vi "AlliGator Compute Phasor Ratio at Mouse Location.vi"(7 "AlliGator Ctrl Refnums":T4, 8 "error in (no error)":errorcluster, 9 "Interactive?":bool, 10 "Mouse Click Event Data":T1, 11 "Data Value Reference in":refnum<data-value>) -> (0 "error out":errorcluster, 1 "Message":string, 3 "Data Value Reference out":refnum<data-value>)   [LabVIEW 2021, in "AlliGator Phasor Ratio.lvlib"]
doc: "Computes phasor ratio and derived quantities at mouse location (interactively or using the last computed phasor) and updates a variety of indicators."
uses:
  AlliGator Phasor Ratio.lvlib
  AlliGator Internal Variables v2.ctl
  <vilib>/vision/Image Controls.llb/IMAQ Image.ctl
  AlliGator Gate Image Set.ctl
  AlliGator FLI Dataset Type.ctl
  AlliGator Data Series Type.ctl
  AlliGator Dataset Channel.ctl
  AlliGator Gate Arithmetic.ctl
  AlliGator Displayed Image.ctl
  Image/Named ROI Description.ctl
  AlliGator Decay Metadata v3.ctl
  AlliGator Decay Background Subtraction Info.ctl
  AlliGator Baseline Subtraction Method.ctl
  Graphs/XY Graph/XY Graph Plot Shift Parameters.ctl
  Graphs/XY Graph/XY Graph Plot Shift Method.ctl
  AlliGator Decay Extrapolation Parameters.ctl
  Phasor/Calibration Phasor (m, phi).ctl
  Phasor/Phasor Reference Series.ctl
  Phasor/Phasor Calibration Map v2.ctl
  Phasor/Phasor (g, s).ctl
  AlliGator Raw Phasor Plot Data v4.ctl
  Phasor/Phasor Standard Deviation Options.ctl
  AlliGator Phasor Multi-Harmonic Data.ctl
  Phasor/Phasor Harmonic Data.ctl
  AlliGator Decay Fit Options & Parameters v2.ctl
  Fits/IRF(X)PSED/Decay Fit Options v2.ctl
  Fits/Decay Convolution/Decay Model.ctl
  Fits/Residual Type.ctl
  Fits/IRF(X)PSED/Fit Weights Type.ctl
  Fits/Non-linear Fitting Method v2.ctl
  Fits/Fit Calculation Method.ctl
  Fits/Non-linear Fitting Algorithm.ctl
  AlliGator Decay Fit Parameter Constraints 2.ctl
  Fits/IRF(X)PSED/Decay Fit Parameters In List.ctl
  Fits/IRF(X)PSED/MLE Baseline Offset Type.ctl
  AlliGator Decay Preprocessing Parameters.ctl
  Fits/IRF(X)PSED/Decay Fit Parameters & Derived Quantities List.ctl
  AlliGator Ctrl Refnums.ctl
  AlliGator Other Ctrl Refnums.ctl
  AlliGator State Indicator.ctl
  AlliGator Phasor Plot Ctrl Refnums.ctl
  AlliGator Phasor Graph Ctrl Refnums.ctl
  Phasor/Phasor Calibration Type.ctl
  AlliGator Dataset Ctrl Refnums.ctl
  AlliGator Registered Events Ctrl Refnums.ctl
  AlliGator Image Histogram Control Refnums.ctl
  Histograms/Linear Histogram Options.ctl
  Histograms/Histogram Bin Option.ctl
  Histograms/Histogram Bin Position.ctl
  AlliGator Decay Fit Map Control Refnums.ctl
  Graphs/XY Graph/XY Graph Mouse Click Event Data.ctl
  Graphs/XY Graph/XY Graph Refnum.ctl
  <vilib>/Utility/miscctls.llb/LVPoint32TypeDef.ctl
  AlliGator Phasor Ratio Parameters.ctl
  Phasor/Phasor (m, phi).ctl
  Phasor/Phasor.lvlib
  AlliGator Intensity Corrections.lvlib
  Graphs/XY Graph/XY Graph Add-Ons.lvlib
  Image/Image.lvlib
  AlliGator Decay Preprocessing.lvlib
  AlliGator Phasor Graph.lvlib
  AlliGator Files.lvlib
  AlliGator Internal Variables.lvlib
  AlliGator Phasor Plot.lvlib
  AlliGator Source Image.lvlib
  Fits/Fits.lvlib
  AlliGator Decay Fit.lvlib
  AlliGator Decay Fit Parameter Map.lvlib
  AlliGator Settings.lvlib
  AlliGator GUI.lvlib
  AlliGator Dual-Channel Datasets.lvlib
  Histograms/Histogram Window.lvlib
panel:
  # "see the AlliGator License on the block diagram (Ctrl+E or Window:Show Block Diagram)"
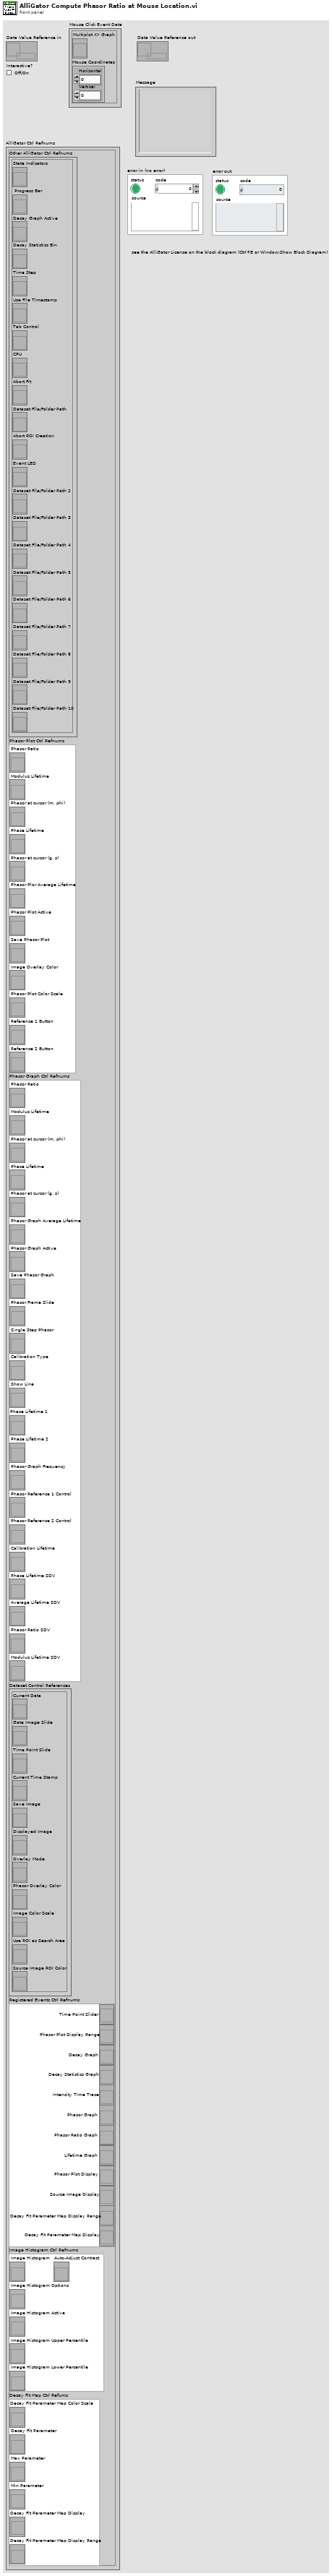
[diagram p1: front panel]
types:
  T1 = typedef "XY Graph Add-Ons.lvlib/XY Graph Mouse Click Event Data.ctl" = cluster{"Multiplot XY Graph":T2, "Mouse Coordinates":T3}
  T2 = typedef "XY Graph Add-Ons.lvlib/XY Graph Refnum.ctl" = refnum<vi>
  T3 = typedef "LVPoint32TypeDef.ctl" = cluster{"Horizontal":i32, "Vertical":i32}
  T4 = typedef "AlliGator GUI.lvlib/AlliGator Ctrl Refnums.ctl" = cluster{"Other AlliGator Ctrl Refnums":T5, "Phasor Plot Ctrl Refnums":T6, "Phasor Graph Ctrl Refnums":T7, "Dataset Control References":T8, "Registered Events Ctrl Refnums":T9, "Image Histogram Ctrl Refnums":T10, "Decay Fit Map Ctrl Refums":T11}
  T5 = typedef "AlliGator GUI.lvlib/AlliGator Other Ctrl Refnums.ctl" = cluster{"State Indicators":refnum<vi>, " Progress Bar":refnum<vi>, "Decay Graph Active":refnum<vi>, "Decay Statistics Bin":refnum<vi>, "Time Step":refnum<vi>, "Use File Timestamp":refnum<vi>, "Tab Control":refnum<vi>, "CPU":refnum<vi>, "Abort Fit":refnum<vi>, "Dataset File/Folder Path":refnum<vi>, "Abort ROI Creation":refnum<vi>, "Event LED":refnum<vi>, "Dataset File/Folder Path 2":refnum<vi>, "Dataset File/Folder Path 3":refnum<vi>, "Dataset File/Folder Path 4":refnum<vi>, "Dataset File/Folder Path 5":refnum<vi>, "Dataset File/Folder Path 6":refnum<vi>, "Dataset File/Folder Path 7":refnum<vi>, "Dataset File/Folder Path 8":refnum<vi>, "Dataset File/Folder Path 9":refnum<vi>, "Dataset File/Folder Path 10":refnum<vi>}
  T6 = typedef "AlliGator GUI.lvlib/AlliGator Phasor Plot Ctrl Refnums.ctl" = cluster{"Phasor Ratio":refnum<vi>, "Modulus Lifetime":refnum<vi>, "Phasor at cursor (m, phi)":refnum<vi>, "Phase Lifetime":refnum<vi>, "Phasor at cursor (g, s)":refnum<vi>, "Phasor Plor Average Lifetime":refnum<vi>, "Phasor Plot Active":refnum<vi>, "Save Phasor Plot":refnum<vi>, "Image Overlay Color":refnum<vi>, "Phasor Plot Color Scale":refnum<vi>, "Reference 1 Button":refnum<vi>, "Reference 2 Button":refnum<vi>}
  T7 = typedef "AlliGator GUI.lvlib/AlliGator Phasor Graph Ctrl Refnums.ctl" = cluster{"Phasor Ratio":refnum<vi>, "Modulus Lifetime":refnum<vi>, "Phasor at cursor (m, phi)":refnum<vi>, "Phase Lifetime":refnum<vi>, "Phasor at cursor (g, s)":refnum<vi>, "Phasor Graph Average Lifetime":refnum<vi>, "Phasor Graph Active":refnum<vi>, "Save Phasor Graph":refnum<vi>, "Phasor Frame Slide":refnum<vi>, "Single Step Phasor":refnum<vi>, "Calibration Type":refnum<vi>, "Show Line":refnum<vi>, "Phase Lifetime 1":refnum<vi>, "Phase Lifetime 2":refnum<vi>, "Phasor Graph Frequency":refnum<vi>, "Phasor Reference 1 Control":refnum<vi>, "Phasor Reference 2 Control":refnum<vi>, "Calibration Lifetime":refnum<vi>, "Phase Lifetime SDV":refnum<vi>, "Average Lifetime SDV":refnum<vi>, "Phasor Ratio SDV":refnum<vi>, "Modulus Lifetime SDV":refnum<vi>}
  T8 = typedef "AlliGator GUI.lvlib/AlliGator Dataset Ctrl Refnums.ctl" = cluster{"Current Data":refnum<vi>, "Gate Image Slide":refnum<vi>, "Time Point Slide":refnum<vi>, "Current Time Stamp":refnum<vi>, "Save Image":refnum<vi>, "Displayed Image":refnum<vi>, "Overlay Mode":refnum<vi>, "Phasor Overlay Color":refnum<vi>, "Image Color Scale":refnum<vi>, "Use ROI as Search Area":refnum<vi>, "Source Image ROI Color":refnum<vi>}
  T9 = typedef "AlliGator GUI.lvlib/AlliGator Registered Events Ctrl Refnums.ctl" = cluster{"Time Point Slider":refnum<vi>, "Phasor Plot Display Range":refnum<vi>, "Decay Graph":refnum<vi>, "Decay Statistics Graph":refnum<vi>, "Intensity Time Trace":refnum<vi>, "Phasor Graph":refnum<vi>, "Phasor Ratio Graph":refnum<vi>, "Lifetime Graph":refnum<vi>, "Phasor Plot Display":refnum<vi>, "Source Image Display":refnum<vi>, "Decay Fit Parameter Map Display Range":refnum<vi>, "Decay Fit Parameter Map Display":refnum<vi>}
  T10 = typedef "AlliGator GUI.lvlib/AlliGator Image Histogram Control Refnums.ctl" = cluster{"Image Histogram":refnum<vi>, "Image Histogram Options":refnum<vi>, "Image Histogram Active":refnum<vi>, "Image Histogram Upper Percentile":refnum<vi>, "Image Histogram Lower Percentile":refnum<vi>, "Auto-Adjust Contrast":refnum<vi>}
  T11 = typedef "AlliGator Decay Fit Parameter Map.lvlib/AlliGator Decay Fit Map Control Refnums.ctl" = cluster{"Decay Fit Parameter Map Color Scale":refnum<vi>, "Decay Fit Parameter":refnum<vi>, "Max Parameter":refnum<vi>, "Min Parameter":refnum<vi>, "Decay Fit Parameter Map Display":refnum<vi>, "Decay Fit Parameter Map Display Range":refnum<vi>}
  T12 = typedef "AlliGator Phasor Ratio.lvlib/AlliGator Phasor Ratio Parameters.ctl" = cluster{"Calibrated Phasor Series":T13[], "Last Calibrated Phasor":T13, "Phasor Ratio Reference 1":T13, "Reference Lifetime 1":dbl[unit], "Phasor Ratio Reference 2":T13, "Reference Lifetime 2":dbl[unit], "Reference Decay":cluster{"t Array":dbl[], "I Array":dbl[]}, "Last Calibrated Phasor SDV":T13}
  T13 = typedef "Phasor.lvlib/Phasor (g, s).ctl" = cluster{"g":dbl, "s":dbl}
  T14 = typedef "Phasor.lvlib/Phasor (m, phi).ctl" = cluster{"m":dbl, "phi":dbl}
  T15 = typedef "AlliGator Internal Variables.lvlib/AlliGator Internal Variables v2.ctl" = cluster{"Displayed Image":T16, "White Light Image":T16, "Mask Image":T16, "ROI Mask Image":T16, "Current Dataset Images 1":T17, "Background Dataset Images 1":T17, "Current Dataset Images 2":T17, "Background Dataset Images 2":T17, "Current Dataset Arithmetic Images":T17, "Accumulated Dataset Images 1":T17, "Accumulated Dataset Images 2":T17, "Accumulated Dataset Arithmetic Images":T17, "Phasor Plot Image":T16, "Decay Fit Parameter Map Image":T16, "Single Data Point Path":path, "White Light Image Path":path, "Mask Image Path":path, "Time-Series Folder":path, "[Time-Series Paths]":path[], "Current Dataset":i32, "Single Dataset Type":T18, "Current Folder":string, "AlliGator Data Series Type":T19, "# Datasets":i32, "Dual-Channel Dataset":bool, "Selected Channel Name":string, "Dataset Channel":T20, "Channel Arithmetic":T21, "Dual-Channel Background Dataset":bool, "Background Channel":T20, "Dual-Channel Accumulated Dataset":bool, "Start Time":dbl, "[Time-Series Timestamps]":dbl[], "[Intensity Corrections]":dbl[], "Time Series Script":bool, "Type of Displayed Image":T22, "Gate Image Slide":u16, "# Gates":i32, "ROIs":T23[], "ROI Decay":cluster{"t Array":dbl[], "I Array":dbl[]}, "Valid Decay":bool, "Decay  Metadata":T25, "Reference Decay Plot Name":string, "Reference Decay":cluster{"t Array":dbl[], "I Array":dbl[]}, "Decay Shift Plot":cluster{"Time Stamps":dbl[], "Decay Shifts":dbl[]}, "[Decays Max Values]":sgl[], "[Decays Min Values]":sgl[], "Calibration Phasor":T31, "Calibration Phasor Series":T32, "Phasor Calibration Map":T33, "Calibration Map MD5 Digest":string, "Last Raw Phasor":T13, "Last Calibrated Phasor":T13, "Last Calibrated Phasor SDV":T13, "Phasor Graph:Phasor Plot":cluster{"g Array":dbl[], "s Array":dbl[]}, "Phasor Graph:Phasor SDV Plot":cluster{"g Array":dbl[], "s Array":dbl[]}, "[Phasor Graph:Raw Phasor Plots]":T34[], "Phasor Plot locked to Ref 1":i32, "[Phasor Plot(s) locked to Ref 1]":i32[], "[Phasor Plot(s) locked to Ref 2]":i32[], "[Pixel Phasors]":T13[], "[[Sum Image]]":dbl[][], "[[CSG Phasors]]":csg[][], "[[Valid Pixel?]]":bool[][], "I/m/phi Dataset":cluster{"I/m/phi Dataset?":bool, "Base Frequency":dbl[unit], "Harmonic Orders":u8[]}, "Multi Phasor Plot Data":T36, "Decay Fit Options & Parameters":T38, "Fit Options: Decay Preprocessing Parameters":T49, "Fit Options: Reference Decay":cluster{"t Array":dbl[], "I Array":dbl[]}, "Is Full Image Parameters Map":bool, "Is Single-Pixels Parameters Map":bool, "NLSF Parameters Map X Resolution":i32, "NLSF Parameters Map Y Resolution":i32, "[Single Decay Fit Parameters]":dbl[], "Fit Model":T40, "[[Multiple Decays Fit Parameters]]":dbl[][], "[[Multiple Decays Fit Parameter SDVs]]":dbl[][], "[[IRFs]]":dbl[][], "IRF Array Time Axis":dbl[], "Decay Array Time Axis":dbl[], "[Decay Fit Parameter Names]":T50[], "[[Phasor Ratios]]":dbl[][], "[[Average Lifetimes]]":dbl[][], "Amplitude Weighted Average Lifetime":bool, "[Decay Sum]":dbl[], "[[User-defined Quantities]]":dbl[][], "User-defined Quantity":string}
  T16 = typedef "IMAQ Image.ctl" = refnum<image>
  T17 = typedef "AlliGator Internal Variables.lvlib/AlliGator Gate Image Set.ctl" = cluster{"SGL Image Max":T16, "SGL Image Sum":T16, "SGL Gate Images":T16[], "SGL Image Min":T16}
  T18 = typedef "AlliGator Files.lvlib/AlliGator FLI Dataset Type.ctl" = enum16{"HDF5 FLI Dataset", "Gate Image Folder", ".sdt FLI Dataset (Becker & Hickl)", ".ptu FLI Dataset (PicoQuant)", "SS1 FLI Dataset", "SS2 FLI Dataset", "I/m/phi Dataset", ".bin FLI Dataset (PicoQuant Binned)", ".bin FLI Dataset (Piccolo Binned)"}
  T19 = typedef "AlliGator Files.lvlib/AlliGator Data Series Type.ctl" = enum16{"Not a Supported Series", "Gate Images Folder Series", "SwissSPAD 2 Dataset Series", "B&H FLI Dataset Series", "PicoQuant PTU FLI Dataset Series", "PicoQuant BIN FLI Dataset Series", "Piccolo hist BIN FLI Dataset Series", "HDF5 FLI Dataset Series"}
  T20 = typedef "AlliGator Dual-Channel Datasets.lvlib/AlliGator Dataset Channel.ctl" = enum16{"G2", "INT"}
  T21 = typedef "AlliGator Settings.lvlib/AlliGator Gate Arithmetic.ctl" = enum16{"None", "INT-G2", "G2/INT*<INT>", "(1 - G2/INT)*<INT>"}
  T22 = typedef "AlliGator Source Image.lvlib/AlliGator Displayed Image.ctl" = enum16{"Single Gate", "Sum of All Gates", "Max of All Gates", "Min of All Gates", "-", "White Ligth Image", "Mask Image"}
  T23 = typedef "Image.lvlib/Named ROI Description.ctl" = cluster{"ROI Descriptor":T24, "ROI Name":string, "Overlay Color":u32}
  T24 = typedef "ROI Descriptor" = cluster{"Global Rectangle":i32[], "Contours":cluster{"ID":enum32{"External", "Internal"}, "Type":u32, "Coordinates":i32[]}[]}
  T25 = typedef "AlliGator Phasor Graph.lvlib/AlliGator Decay Metadata v3.ctl" = cluster{"ROI Descriptor":T24, "ROI Center":cluster{"X":i32, "Y":i32}, "Decay Background Subtraction Info":T26, "Decay Reverted":bool, "Decay Smoothened":bool, "Decay Straightened":bool, "Fitted Tau (Decay Straightening)":dbl, "Decay Shift Parameters":T28, "Decay Shifted":bool, "Decay Extrapolated":bool, "Decay Extrapolation Parameters":T30, "Decay Normalized":bool, "Fold Decay":bool, "# Folds":u32}
  T26 = typedef "AlliGator Decay Analysis.lvlib/AlliGator Decay Preprocessing.lvlib/AlliGator Decay Background Subtraction Info.ctl" = cluster{"Laser Period":dbl[unit], "Gate Duration":dbl[unit], "Baseline Subtraction Method":T27, "Background Definition Range":cluster{"Min Gate":dbl[unit], "Max Gate":dbl[unit]}, "Total Intensity w/o Bkgd Subtraction":dbl, "Bkgd-subtracted Intensity (exp)":dbl, "# Data Points":i32, "Background/Gate":dbl, "Fitted Lifetime":dbl[unit], "Bkgd-subtracted Intensity (theo)":dbl}
  T27 = typedef "AlliGator Decay Analysis.lvlib/AlliGator Decay Preprocessing.lvlib/AlliGator Baseline Subtraction Method.ctl" = enum16{"Mean", "Min", "Square Gated Single-Exponential", "File", "Constant"}
  T28 = typedef "XY Graph Add-Ons.lvlib/XY Graph Plot Shift Parameters.ctl" = cluster{"Type":T29, "Shift":dbl[unit], "Threshold":dbl, "Rotate":bool}
  T29 = typedef "XY Graph Add-Ons.lvlib/XY Graph Plot Shift Method.ctl" = enum16{"Default", "CFD", "Threshold", "Cross-Correlation"}
  T30 = typedef "AlliGator Decay Analysis.lvlib/AlliGator Decay Preprocessing.lvlib/AlliGator Decay Extrapolation Parameters.ctl" = cluster{"Additional Points":u32, "Head Fraction":dbl, "Fitted Tau":dbl, "Use Periodicity":bool, "Use Cursors":bool, "Tail Fraction":dbl}
  T31 = typedef "Phasor.lvlib/Calibration Phasor (m, phi).ctl" = cluster{"m":dbl, "phi":dbl, "Phasor Frequency":dbl[unit], "Reference Lifetime":dbl[unit]}
  T32 = typedef "Phasor.lvlib/Phasor Reference Series.ctl" = cluster{"m Array":dbl[], "phi Array":dbl[], "Phasor Frequency":dbl[unit], "Calibration Lifetime":dbl[unit]}
  T33 = typedef "Phasor.lvlib/Phasor Calibration Map v2.ctl" = cluster{"Phasor Frequency":dbl[unit], "Calibration Lifetime":dbl[unit], "ROI Centers":cluster{"X":i32, "Y":i32}[], "ROI Descriptors":T24[], "Map Resolution X":i32, "Map Resolution Y":i32, "z Array":cdb[]}
  T34 = typedef "AlliGator Phasor Graph.lvlib/AlliGator Raw Phasor Plot Data v4.ctl" = cluster{"Phasor Plot Name":string, "Raw Phasor Plot":T13[], "Phasor Frequency":dbl[unit], "[Decay Metadata]":T25[], "Raw Phasor Plot SDV":T13[], "Phasor SDV Options":T35, "[Calibration Phasor]":T31[]}
  T35 = typedef "Phasor.lvlib/Phasor Standard Deviation Options.ctl" = cluster{"Compute Estimated SDV":bool, "# Replicas":u32, "Use Estimated Average Phasor":bool}
  T36 = typedef "AlliGator Phasor Plot.lvlib/AlliGator Phasor Multi-Harmonic Data.ctl" = cluster{"Base Frequency":dbl[unit], "# Harmonics":u8, "Harmonic Orders":u8[], "Phasor Plot Settings Checksum":u64, "Phasor Harmonic Data Array":T37[]}
  T37 = typedef "Phasor.lvlib/Phasor Harmonic Data.ctl" = cluster{"Phasor Harmonic Name":string, "Phasor Plot Settings Checksum":u64, "Phasor Frequency":dbl[unit], "Base Frequency":dbl[unit], "Harmonic Order":u8, "Phasor Plot Parameters":string, "Phasor Array [[CSG]]":csg[][], "Dataset File Path":path}
  T38 = typedef "AlliGator Decay Fit Parameter Map.lvlib/AlliGator Decay Fit Options & Parameters v2.ctl" = cluster{"SYNC Period":dbl[unit], "Fit Options":T39, "Fit Parameter Constraints":T46[], "MLE Baseline Offset":dbl, "MLE Baseline Offset Type":T48}
  T39 = typedef "Fits.lvlib/Decay Fit Options v2.ctl" = cluster{"Show Fit Residuals":bool, "Fit Model":T40, "Residual Type":T41, "Max Decay Percentile":dbl, "Min Decay Percentile":dbl, "Show Full Decay":bool, "Weights":T42, "Fitting Method":T43, "Compute Parameter Uncertainties":bool, "Periodic Boundaries":bool, "Model Calculation":T44, "Period":dbl[unit], "Termination Criteria":cluster{"Max Iterations":i32, "Max Function Calls":i32, "Max Time":dbl[unit], "Function Tolerance":dbl, "Parameter Tolerance":dbl, "Gradient Tolerance":dbl, "Min Lambda":dbl, "Max Lambda":dbl, "Initial Tick Count":u32}, "Offset Resolution":dbl[unit], "Use Local IRF":bool, "Fitting Algorithm":T45}
  T40 = typedef "Fits.lvlib/Decay Model.ctl" = enum16{"1-Exponential", "2-Exponentials"}
  T41 = typedef "Fits.lvlib/Residual Type.ctl" = enum16{"Standard", "Normalized", "Reduced"}
  T42 = typedef "Fits.lvlib/Fit Weights Type.ctl" = enum16{"Unweighted", "1/Variance", "Best of All"}
  T43 = typedef "Fits.lvlib/Non-linear Fitting Method v2.ctl" = enum16{"Least Square", "Least Absolute Residual", "Bisquare", "MLE", "-", "Best of All"}
  T44 = typedef "Fits.lvlib/Fit Calculation Method.ctl" = enum16{"Simulation", "Convolution", "Integration"}
  T45 = typedef "Fits.lvlib/Non-linear Fitting Algorithm.ctl" = enum16{"Levenberg-Marquardt", "Trust-Region Dogleg"}
  T46 = typedef "AlliGator Decay Analysis.lvlib/AlliGator Decay Fit.lvlib/AlliGator Decay Fit Parameter Constraints 2.ctl" = cluster{"Fit Parameter":T47, "Min Value":dbl, "Max Value":dbl, "Global":bool, "Used":bool}
  T47 = typedef "Fits.lvlib/Decay Fit Parameters In List.ctl" = enum16{"Offset", "Baseline", "A_1", "tau_1", "A_2", "tau_2"}
  T48 = typedef "Fits.lvlib/MLE Baseline Offset Type.ctl" = enum32{"Absolute", "Percentage"}
  T49 = typedef "AlliGator Decay Analysis.lvlib/AlliGator Decay Preprocessing.lvlib/AlliGator Decay Preprocessing Parameters.ctl" = cluster{"Background Subtraction":bool, "Straighten Decay":bool, "Reverse Gates":bool, "1-Normalized Decay":bool, "Smoothen Decay":bool, "Smoothing Parameter":dbl, "Shift Decay":bool, "Decay Shift Parameters":T28, "Extrapolate Decay":bool, "Additional Points":u32, "Head Fraction":dbl, "Pixel-Normalize Decay":bool, "Use Periodicity":bool, "Use Cursors":bool, "Tail Fraction":dbl, "Use Decay Pre-Processing":bool, "Fold Decay":bool, "# Folds":u32, "[0-1]-Normalized Decay":bool}
  T50 = typedef "Fits.lvlib/Decay Fit Parameters & Derived Quantities List.ctl" = enum16{"Offset", "Baseline", "A_1", "tau_1", "A_2", "tau_2", "<tau>_a", "f1_a", "f2_a", "<tau>_i", "f1_i", "f2_i", "-", "R^2", "Chi^2"}
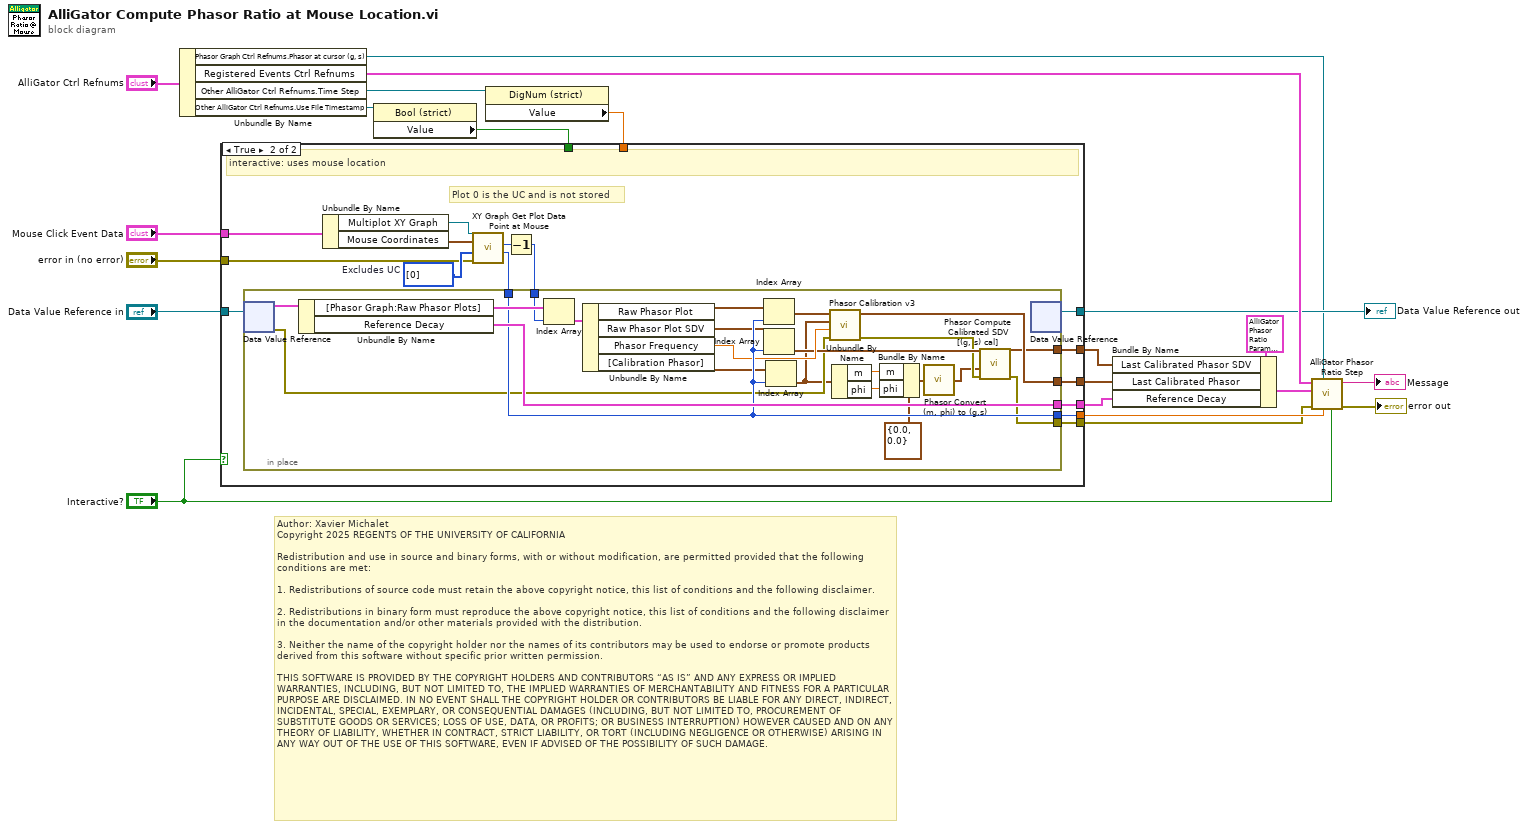
[diagram p0: block diagram]
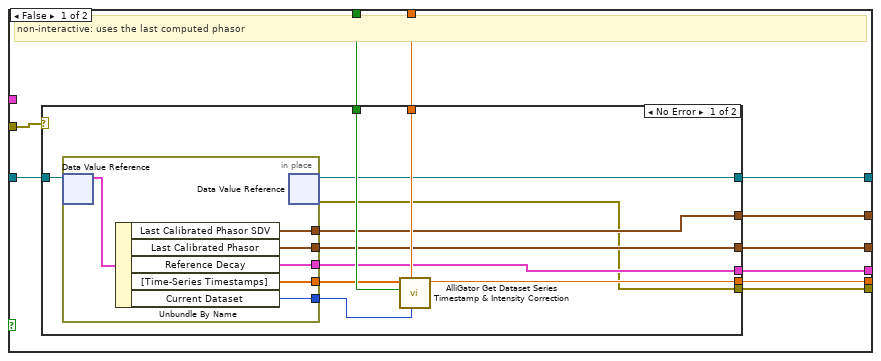
[diagram p2: hidden frame]
diagram:
  # "Author: Xavier Michalet\nCopyright 2025 REGENTS OF THE UNIVERSITY OF CALIFORNIA\n\nRedistribution and use in source and binary forms, with or without modification, are permitted provided that the following conditions are met:\n\n1. Redistributions of source code must retain the above copyright notice, this list of conditions and the following disclaimer.\n\n2. Redistributions in binary form must reproduce the above copyright notice, this list of conditions and the following disclaimer in the documentation and/or other materials provided with the distribution.\n\n3. Neither the name of the copyright holder nor the names of its contributors may be used to endorse or promote products derived from this software without specific prior written permission.\n\nTHIS SOFTWARE IS PROVIDED BY THE COPYRIGHT HOLDERS AND CONTRIBUTORS “AS IS” AND ANY EXPRESS OR IMPLIED WARRANTIES, INCLUDING, BUT NOT LIMITED TO, THE IMPLIED WARRANTIES OF MERCHANTABILITY AND FITNESS FOR A PARTICULAR PURPOSE ARE DISCLAIMED. IN NO EVENT SHALL THE COPYRIGHT HOLDER OR CONTRIBUTORS BE LIABLE FOR ANY DIRECT, INDIRECT, INCIDENTAL, SPECIAL, EXEMPLARY, OR CONSEQUENTIAL DAMAGES (INCLUDING, BUT NOT LIMITED TO, PROCUREMENT OF SUBSTITUTE GOODS OR SERVICES; LOSS OF USE, DATA, OR PROFITS; OR BUSINESS INTERRUPTION) HOWEVER CAUSED AND ON ANY THEORY OF LIABILITY, WHETHER IN CONTRACT, STRICT LIABILITY, OR TORT (INCLUDING NEGLIGENCE OR OTHERWISE) ARISING IN ANY WAY OUT OF THE USE OF THIS SOFTWARE, EVEN IF ADVISED OF THE POSSIBILITY OF SUCH DAMAGE."
  n1 = Unbundle By Name("AlliGator Ctrl Refnums") -> ("Phasor Graph Ctrl Refnums.Phasor at cursor (g, s)"=w2:refnum<vi>, "Registered Events Ctrl Refnums"=w20:T9, "Other AlliGator Ctrl Refnums.Time Step"=w14:refnum<vi>, "Other AlliGator Ctrl Refnums.Use File Timestamp"=w12:refnum<vi>)
  n2 = property class="Bool (strict)"(reference=w12) -> ("Value"=w11:bool)  [unwired: 1 in, 2 out]
  n3 = property class="DigNum (strict)"(reference=w14) -> ("Value"=w13:dbl[unit])  [unwired: 1 in, 2 out]
  n4 = case shown="True" "Interactive?" {
    tunnel: [w31 w62] -> w19
    tunnel: w13 -> [w30 _]
    tunnel: w11 -> [w29 _]
    tunnel: "Data Value Reference in" -> [w28 w65]
    tunnel: [w27 w64] -> w9
    tunnel: [w26 w61] -> w8
    tunnel: [w25 w63] -> w7
    tunnel: [w24 w60] -> w6
    tunnel: "error in (no error)" -> [w22 w51]
    tunnel: "Mouse Click Event Data" -> [_ w52]
    tunnel: [w23 w59] -> w3
    frame False {
      # "non-interactive: uses the last computed phasor"
      n5 = case shown="No Error" w22 {
        selector: w22 -> [_ w49]
        tunnel: [w42 _] -> w31
        tunnel: w30 -> [w41 _]
        tunnel: w29 -> [w40 _]
        tunnel: w28 -> [w39 w50]
        tunnel: [w38 w50] -> w27
        tunnel: [w37 _] -> w26
        tunnel: [w36 _] -> w25
        tunnel: [w33 _] -> w24
        tunnel: [w32 w49] -> w23
        frame No Error {
          n6 = in-place {
            in-place-border: [w47] -> w37
            in-place-border: [w46] -> w36
            in-place-border: [w44] -> w35
            in-place-border: [w43] -> w34
            in-place-border: [w45] -> w33
            n7 = in-place-dvr #1(w39) -> (w48:T15)  [unwired: 1 out]
            n8 = Unbundle By Name(w48) -> ("Last Calibrated Phasor SDV"=w45:T13, "Last Calibrated Phasor"=w47:T13, "Reference Decay"=w46:cluster{"t Array":dbl[], "I Array":dbl[]}, "[Time-Series Timestamps]"=w44:dbl[], "Current Dataset"=w43:i32)
            n9 = in-place-dvr #1() -> (w38:refnum<data-value>, w32:errorcluster)  [unwired: 1 in]
          }
          n10 = call "AlliGator Get Dataset Series Timestamp & Intensity Correction.vi"("Current Data Set"=w34, "Time Step"=w41, "Use File Timestamp"=w40, "Dataset Series Timestamps"=w35) -> ("Time Stamp (s)"=w42:dbl)  [unwired: 6 in, 1 out]
        }
        frame Error {
        }
      }
    }
    frame True {
      w56 = i32[] [0]  # Excludes UC
      # "Plot 0 is the UC and is not stored"
      # "interactive: uses mouse location"
      n11 = Unbundle By Name(w52) -> ("Multiplot XY Graph"=w58:T2, "Mouse Coordinates"=w57:T3)
      n12 = call "XY Graph Get Plot Data Point at Mouse.vi"("Error In"=w51, "Excluded Plots"=w56, "Coords"=w57, "XYGraph in"=w58) -> ("Point  Index"=w54:i32, "Plot Number"=w55:i32)  [unwired: 3 in, 3 out]
      n13 = Decrement(x=w55) -> (x-1=w53:i32)
      n14 = in-place {
        in-place-border: w53 -> [w86]
        in-place-border: [w84] -> w63
        in-place-border: [w81] -> w62
        in-place-border: w54 -> [w81]
        in-place-border: [w77] -> w61
        in-place-border: [w73] -> w60
        in-place-border: [w72] -> w59
        n15 = in-place-dvr #2(w65) -> (w88:T15, w74:errorcluster)
        n16 = Unbundle By Name(w88) -> ("[Phasor Graph:Raw Phasor Plots]"=w87:T34[], "Reference Decay"=w84:cluster{"t Array":dbl[], "I Array":dbl[]})
        n17 = Index Array(array=w87, index=w86) -> (element=w85:T34)
        n18 = Unbundle By Name(w85) -> ("Raw Phasor Plot"=w83:T13[], "Raw Phasor Plot SDV"=w80:T13[], "Phasor Frequency"=w79:dbl[unit], "[Calibration Phasor]"=w78:T31[])
        n19 = Index Array(array=w83, index=w81) -> (element=w82:T13)
        n20 = Index Array(array=w80, index=w81) -> (element=w76:T13)
        n21 = Index Array(array=w78, index=w81) -> (element=w70:T31)
        n22 = call "Phasor Calibration v3.vi"("Error In"=w74, "Phasor Frequency"=w79, "Calibration Phasor"=w70, "Measured Phasor"=w82) -> ("Error Out"=w75:errorcluster, "Calibrated Phasor"=w77:T13)  [unwired: 2 in, 4 out]
        n23 = Unbundle By Name(w70) -> ("m"=w68:dbl, "phi"=w66:dbl)
        n24 = Bundle By Name(cluster=T14 {"m"=0.0, "phi"=0.0} ("Phasor (m, phi)"), "m"=w68, "phi"=w66) -> (w67:T14)
        n25 = call "Phasor Convert (m, phi) to (g,s).vi"("Phasor (m, phi)"=w67) -> ("Phasor (g, s)"=w71:T13)  [unwired: 8 in]
        n26 = call "Phasor Compute Calibrated SDV [(g, s) cal].vi"("Error In"=w75, "Phasor Calibration (g,s)"=w71, "Raw Phasor SDV (g, s)"=w76) -> ("Error Out"=w72:errorcluster, "Calibrated Phasor SDV (g, s)"=w73:T13)  [unwired: 7 in]
        n27 = in-place-dvr #2() -> (w64:refnum<data-value>)  [unwired: 1 in, 1 out]
      }
    }
  }
  "Data Value Reference out" <- w9
  n28 = Bundle By Name(cluster=T12 {"Calibrated Phasor Series"=[], "Last Calibrated Phasor"={"g"=0.0, "s"=0.0}, "Phasor Ratio Reference 1"={"g"=0.0, "s"=0.0}, "Reference Lifetime 1"=0.0, "Phasor Ratio Reference 2"={"g"=0.0, "s"=0.0}, "Reference Lifetime 2"=0.0, "Reference Decay"={"t Array"=[], "I Array"=[]}, "Last Calibrated Phasor SDV"={"g"=0.0, "s"=0.0}} ("Phasor Ratio Parameters"), "Last Calibrated Phasor SDV"=w6, "Last Calibrated Phasor"=w8, "Reference Decay"=w7) -> (w17:T12)
  n29 = call "AlliGator Phasor Ratio Step.vi"("Interactive?"="Interactive?", "Time Stamp"=w19, "Current Phasor Refnum"=w2, "Error In"=w3, "Phasor Ratio Parameters"=w17, "Registered Events Ctrl Refnums"=w20) -> ("Error Out"=→"error out":errorcluster, "Notebook String"=→"Message":string)  [unwired: 4 in]
